vi "Main.vi"() -> ()   [LabVIEW 2017]
uses:
  Program Files/National Instruments/LabVIEW 2019/user.lib/Nanonis Prog Interface V5/Nanonis Prog Interface.lvlib
  <vilib>/ptbypt/NI_PtbyPt.lvlib
panel:
  out "ms/loop":dbl[](array[numeric])
  out "Z position (m)":sgl format="%#_6p"
  out "Current (A)":sgl format="%#_6p"
  in  "Iterations":i32=1000
  # "Testing if Nanonis hates LabVIEW"
  # ":)"
  # "Key:\n0: Current\n1: Z pos Read\n2: XY Move\n3: Z pos Write"
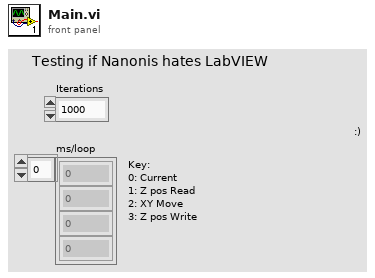
[diagram p1: front panel]
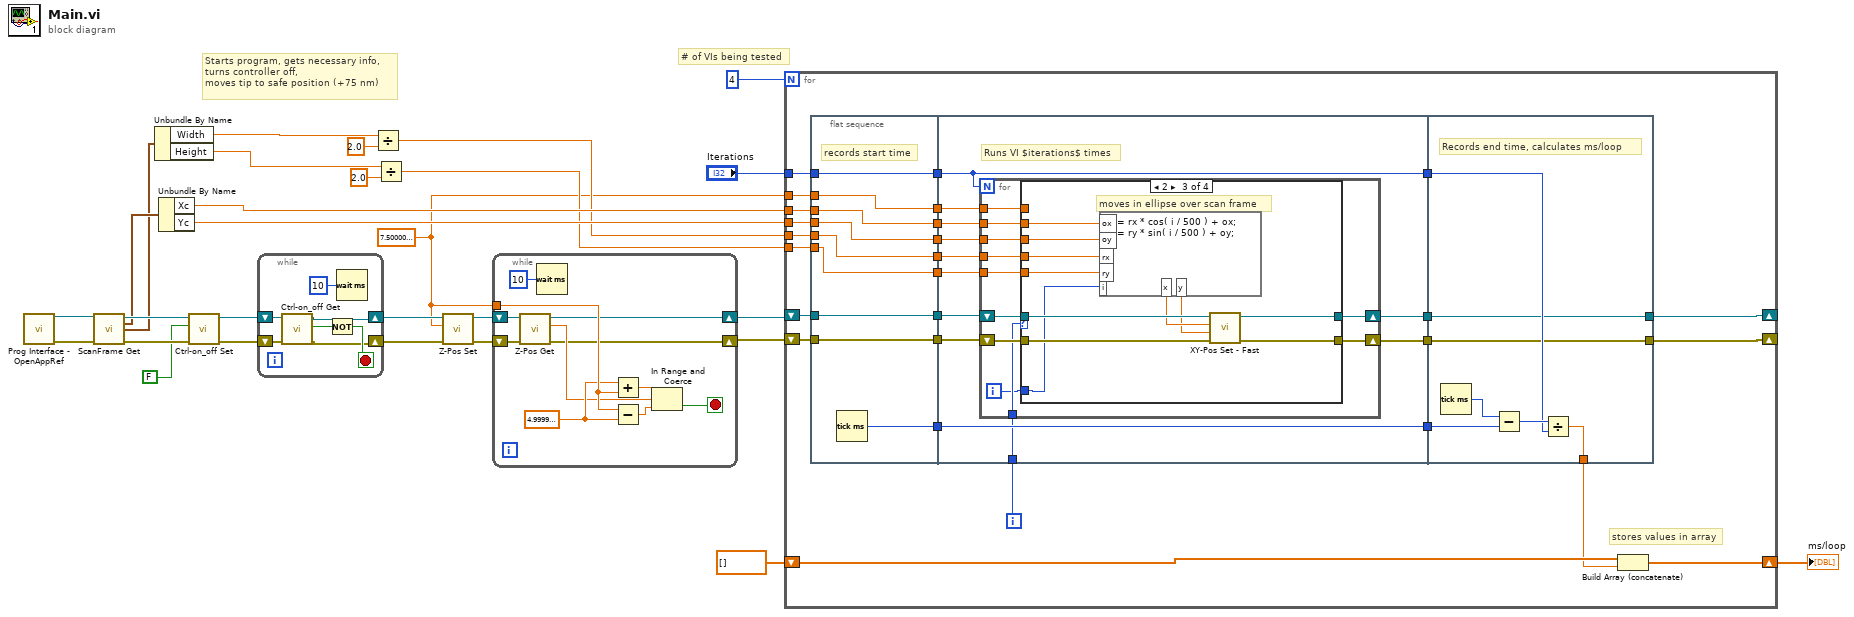
[diagram p0: block diagram]
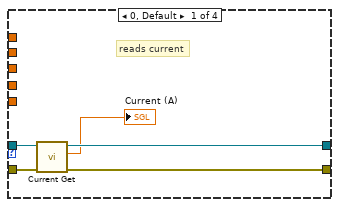
[diagram p2: hidden frame]
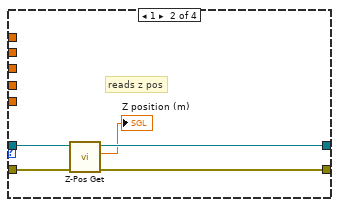
[diagram p3: hidden frame]
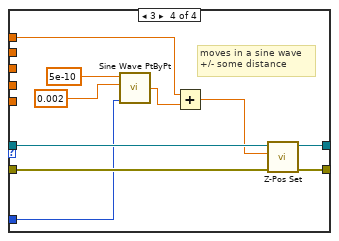
[diagram p4: hidden frame]
diagram:
  w1 = sgl 7.5e-08 ("Z position (m)")
  # "# of VIs being tested"
  # "Starts program, gets necessary info,\nturns controller off,\nmoves tip to safe position (+75 nm)"
  n1 = call <userlib>:"Prog Interface - OpenAppRef.vi"() -> ("Error out"=w24:errorcluster, "Application reference"=w25:refnum<vi>)  [unwired: 6 in]
  n2 = call <userlib>:"ScanFrame Get.vi"("Application ref in"=w25, "error in (no error)"=w24) -> ("Application ref out"=w22:refnum<vi>, "Center coordinates (m)"=w11:cluster{"Xc":sgl, "Yc":sgl}, "Size (m)"=w8:cluster{"Width":sgl, "Height":sgl}, "error out"=w21:errorcluster)  [unwired: 9 in, 1 out]
  n3 = Unbundle By Name(w8) -> ("Width"=w7:sgl, "Height"=w3:sgl)
  n4 = Unbundle By Name(w11) -> ("Xc"=w10:sgl, "Yc"=w9:sgl)
  n5 = call <userlib>:"Ctrl-on_off Set.vi"("error in (no error)"=w21, "Z Controller ON/OFF"=FALSE, "Application ref in"=w22) -> ("error out"=w18:errorcluster, "Application ref out"=w19:refnum<vi>)  [unwired: 7 in]
  n6 = while {
    shift-right: [w30] -> w17
    shift-left: w18 -> [w33]
    shift-right: [w31] -> w16
    shift-left: w19 -> [w32]
    stop <- w35 stop-if-true
    n7 = call <userlib>:"Ctrl-on_off Get.vi"("error in (no error)"=w33, "Application ref in"=w32) -> ("error out"=w30:errorcluster, "Z-Controller on/off status"=w29:bool, "Application ref out"=w31:refnum<vi>)  [unwired: 7 in]
    n8 = Not(x=w29) -> (.not. x?=w35:bool)
    n9 = Wait (ms)(milliseconds to wait=u32 10) -> ()  [unwired: 1 out]
  }
  n10 = Divide(x=w7, y=sgl 2.0) -> (x/y=w6:sgl)
  n11 = Divide(x=w3, y=sgl 2.0) -> (x/y=w2:sgl)
  n12 = call <userlib>:"Z-Pos Set.vi"("error in (no error)"=w17, "Z position (m)"=w1, "Application ref in"=w16) -> ("error out"=w14:errorcluster, "Application ref out"=w15:refnum<vi>)  [unwired: 7 in]
  n13 = while {
    shift-right: [w36] -> w12
    shift-left: w14 -> [w44]
    shift-right: [w37] -> w13
    shift-left: w15 -> [w45]
    tunnel: w1 -> [w41]
    stop <- w39 stop-if-true
    w40 = sgl 5e-10 ("x")
    n14 = call <userlib>:"Z-Pos Get.vi"("error in (no error)"=w44, "Application ref in"=w45) -> ("error out"=w36:errorcluster, "Z position (m)"=w38:sgl, "Application ref out"=w37:refnum<vi>)  [unwired: 7 in]
    n15 = Wait (ms)(milliseconds to wait=u32 10) -> ()  [unwired: 1 out]
    n16 = Add(x=w40, y=w41) -> (x+y=w43:sgl)
    n17 = Subtract(x=w41, y=w40) -> (x-y=w42:sgl)
    n18 = In Range and Coerce(upper limit=w43, x=w38, lower limit=w42) -> (In Range?=w39:bool)  [unwired: 1 out]
  }
  n19 = for {
    N: 4 -> [_]
    tunnel: "Iterations" -> [w64]
    shift-right: [w58] -> w23
    shift-left: dbl[] [] -> [w63]
    shift-right: [w62] -> _
    shift-left: w13 -> [w65]
    shift-right: [w60] -> _
    shift-left: w12 -> [w66]
    tunnel: w10 -> [w55]
    tunnel: w9 -> [w54]
    tunnel: w6 -> [w51]
    tunnel: w2 -> [w49]
    tunnel: w1 -> [w48]
    i -> [w67]
    # "stores values in array"
    n20 = flat-sequence {
      tunnel: [w82] -> w73
      tunnel: [w81] -> w72
      tunnel: [w80] -> w71
      tunnel: [w79] -> w70
      tunnel: w64 -> [w82]
      tunnel: w65 -> [w81]
      tunnel: w66 -> [w80]
      tunnel: [w78] -> w56
      tunnel: w55 -> [w78]
      tunnel: w54 -> [w77]
      tunnel: [w77] -> w53
      tunnel: [w76] -> w52
      tunnel: w51 -> [w76]
      tunnel: [w75] -> w50
      tunnel: w49 -> [w75]
      tunnel: w48 -> [w74]
      tunnel: [w74] -> w47
      tunnel: w73 -> [w91]
      tunnel: w72 -> [w94]
      tunnel: w71 -> [w93]
      tunnel: w70 -> [w92]
      tunnel: [w92] -> w69
      tunnel: [w91] -> w68
      tunnel: w67 -> [w90]
      tunnel: [w89] -> w61
      tunnel: [w88] -> w59
      tunnel: w56 -> [w87]
      tunnel: w53 -> [w86]
      tunnel: w52 -> [w85]
      tunnel: w50 -> [w84]
      tunnel: w47 -> [w83]
      tunnel: w69 -> [w142]
      tunnel: w68 -> [w140]
      tunnel: [w139] -> w62
      tunnel: w61 -> [w139]
      tunnel: [w138] -> w60
      tunnel: w59 -> [w138]
      tunnel: [w137] -> w57
      frame #0 {
        # "records start time"
        n21 = Tick Count (ms)() -> (millisecond timer value=w79:u32)
      }
      frame #1 {
        # "Runs VI $iterations$ times"
        n22 = for {
          N: w91 -> [_]
          shift-right: [w102] -> w88
          shift-left: w93 -> [w104]
          shift-right: [w103] -> w89
          shift-left: w94 -> [w105]
          tunnel: w90 -> [w101]
          tunnel: w87 -> [w100]
          tunnel: w86 -> [w99]
          tunnel: w85 -> [w98]
          tunnel: w84 -> [w96]
          tunnel: w83 -> [w95]
          i -> [w97]
          n23 = case shown="2" w101 {
            tunnel: w105 -> [w110 w115 w126 w136]
            tunnel: w104 -> [w109 w114 w125 w135]
            tunnel: [w107 w112 w124 w133] -> w103
            tunnel: [w108 w113 w123 w134] -> w102
            tunnel: w100 -> [_ _ w120 _]
            tunnel: w99 -> [_ _ w119 _]
            tunnel: w98 -> [_ _ w118 _]
            tunnel: w97 -> [_ _ w117 w127]
            tunnel: w96 -> [_ _ w116 _]
            tunnel: w95 -> [_ _ _ w129]
            frame 0, Default {
              # "reads current"
              n24 = call <userlib>:"Current Get.vi"("Error in (no error)"=w109, "Application ref in"=w110) -> ("Error out"=w108:errorcluster, "Current (A)"=→"Current (A)":sgl, "Application ref out"=w107:refnum<vi>)  [unwired: 5 in]
            }
            frame 1 {
              # "reads z pos"
              n25 = call <userlib>:"Z-Pos Get.vi"("error in (no error)"=w114, "Application ref in"=w115) -> ("error out"=w113:errorcluster, "Z position (m)"=→"Z position (m)":sgl, "Application ref out"=w112:refnum<vi>)  [unwired: 7 in]
            }
            frame 2 {
              # "moves in ellipse over scan frame"
              n26 = formula code="x = rx * cos( i / 500 ) + ox;\ny = ry * sin( i / 500 ) + oy;"("rx"=w118, "i"=w117, "oy"=w119, "ox"=w120, "ry"=w116) -> ("x"=w122:dbl, "y"=w121:dbl)
              n27 = call <userlib>:"XY-Pos Set - Fast.vi"("error in (no error)"=w125, "Y (m)"=w121, "X (m)"=w122, "Application ref in"=w126) -> ("error out"=w123:errorcluster, "Application ref out"=w124:refnum<vi>)  [unwired: 5 in]
            }
            frame 3 {
              # "moves in a sine wave \n+/- some distance"
              n28 = call <vilib>:"Sine Wave PtByPt.vi"("time"=w127, "frequency"=0.002, "amplitude"=5e-10) -> ("sine wave"=w130:dbl)  [unwired: 1 in]
              n29 = Add(x=w129, y=w130) -> (x+y=w128:dbl)
              n30 = call <userlib>:"Z-Pos Set.vi"("error in (no error)"=w135, "Z position (m)"=w128, "Application ref in"=w136) -> ("error out"=w134:errorcluster, "Application ref out"=w133:refnum<vi>)  [unwired: 7 in]
            }
          }
        }
      }
      frame #2 {
        # "Records end time, calculates ms/loop"
        n31 = Tick Count (ms)() -> (millisecond timer value=w143:u32)
        n32 = Subtract(x=w143, y=w142) -> (x-y=w141:u32)
        n33 = Divide(x=w141, y=w140) -> (x/y=w137:dbl)
      }
    }
    n34 = Build Array (concatenate)(w63, w57) -> (w58:dbl[])
  }
  "ms/loop" <- w23
